vi "CAN Write.vi"(2 "Interface:CAN:Termination":u32(ring) items=["Off", "On"], 3 "data":T1[](array[typedef]) {"payload" format="%x"; "timestamp" format="%<%.7X\n%x>T"; "type" items=["CAN Data"=0, "CAN Remote"=1, "CAN Bus Error"=2, "CAN 2.0 Data"=8, "CAN FD Data"=16, "CAN FD+BRS Data"=24, "J1939 Data"=192, "Delay"=224, "Log Trigger"=225, "Start Trigger"=226]; "identifier" format="%x"}, 4 "interface":refnum<k21>) -> ()   [LabVIEW 2022 SP3]
uses:
  <vilib>/xnet/xnet.llb/XNET Frame CAN.ctl
  <vilib>/xnet/xnet.llb/XNET Frame Type CAN.ctl
  <vilib>/xnet/xnet.llb/XNET Create Session (Frame Output Stream).vi
  <vilib>/xnet/xnet.llb/XNET Write (Frame CAN).vi
  <resource>/objmgr/xnet.rc
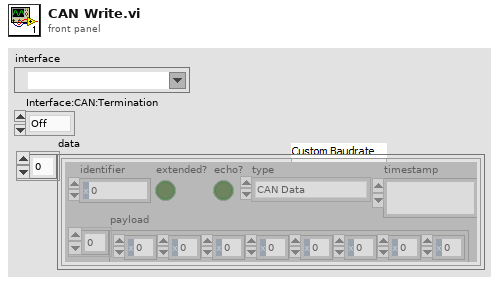
[diagram p1: front panel]
types:
  T1 = typedef "XNET Frame CAN.ctl" = cluster{"timestamp":timestamp, "payload":u8[], "identifier":u32, "type":T2, "extended?":bool, "echo?":bool}
  T2 = typedef "XNET Frame Type CAN.ctl" = u8
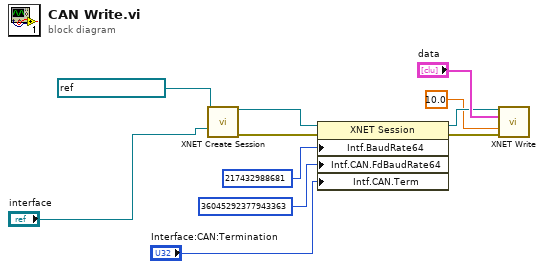
[diagram p0: block diagram]
diagram:
  n1 = call-poly <vilib>:"XNET Create Session.vi"("cluster (:memory:)"=refnum<k21> "Elatch_Labview", "interface"="interface") -> ("session out"=w11:refnum<k21>, "error out"=w10:errorcluster)  [unwired: 12 in]
  n2 = property class="XNET Session"(reference=w11, error in=w10, "Intf.BaudRate64"=u64 217432988681 ("Interface:64bit Baud Rate"), "Intf.CAN.FdBaudRate64"=u64 36045292377943363 ("Interface:CAN:64bit FD Baud Rate"), "Intf.CAN.Term"="Interface:CAN:Termination") -> (reference out=w4:refnum<k21>, error out=w2:errorcluster)
  n3 = call-poly <vilib>:"XNET Write.vi"("session in"=w4, "data"="data", "timeout (10)"=10.0, "error in (no error)"=w2) -> ()  [unwired: 10 in, 2 out]
